vi "Write System Error To DB.vi"(8 "error in (no error)":errorcluster, 10 "Error_Payload":T1, 11 "Refnum in":T2) -> (0 "error out":errorcluster, 3 "Refnum out":T2)   [LabVIEW 2026, in "Database.lvlib"]
uses:
  Database.lvlib
  <vilib>/addons/database/Connection.llb/Conn ObjectReference.ctl
  controls/Diagnostics/Error_Payload.ctl
  <vilib>/addons/database/Connection.llb/Conn Execute.vi
  <vilib>/addons/database/Recordset.llb/Rec Destroy - Connection.vi
  <vilib>/addons/database/NI_Database_API.lvlib
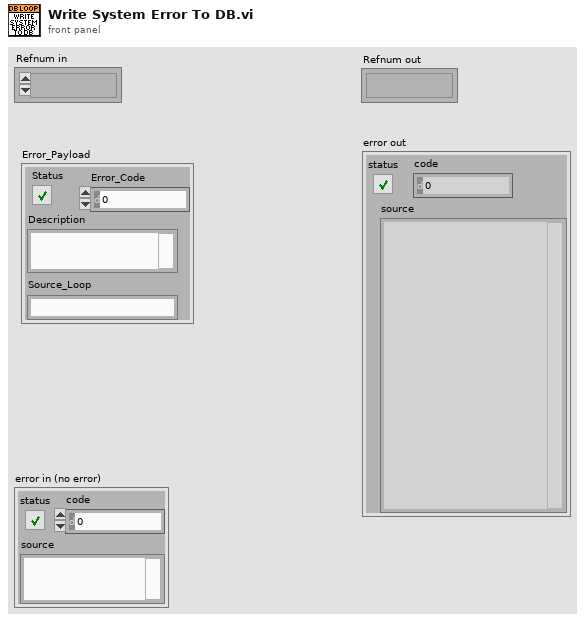
[diagram p1: front panel]
types:
  T1 = typedef "Error_Payload.ctl" = cluster{"status":bool, "error_code":i32, "description":string, "source_loop":string}
  T2 = typedef "NI_Database_API.lvlib/Conn ObjectReference.ctl" = refnum<k1>
  T3 = typedef "NI_Database_API.lvlib/Rec ObjectReference.ctl" = refnum<k1>
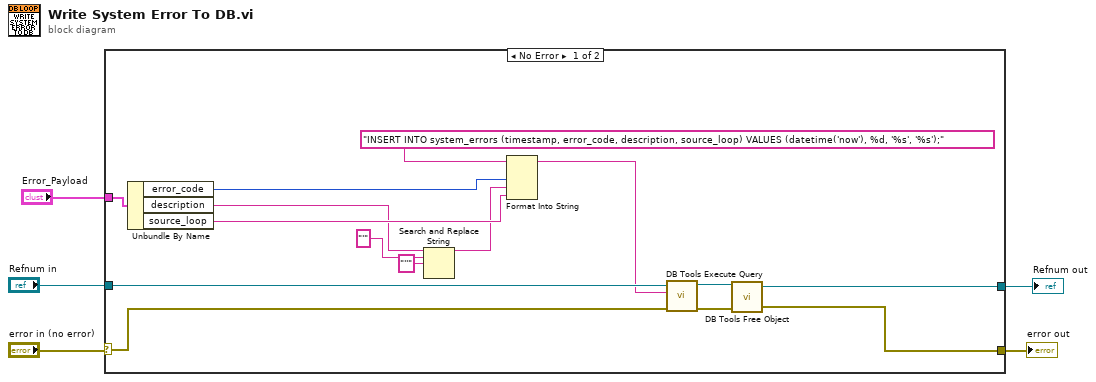
[diagram p0: block diagram]
diagram:
  n1 = case shown="No Error" "error in (no error)" {
    selector: "error in (no error)" -> [w18 w22]
    tunnel: [w16 w22] -> w5
    tunnel: [w17 w21] -> w4
    tunnel: "Refnum in" -> [w19 w21]
    tunnel: "Error_Payload" -> [w20 _]
    frame No Error {
      n2 = Unbundle By Name(w20) -> ("error_code"=w7:i32, "description"=w10:string, "source_loop"=w11:string)
      n3 = Search and Replace String(input string=w10, search string="'" ("format string"), replace string="''" ("replace string (\"\")")) -> (result string=w6:string)  [unwired: 5 in, 3 out]
      n4 = Format Into String(format string="INSERT INTO system_errors (timestamp, error_code, description, source_loop) VALUES (datetime('now'), %d, '%s', '%s');", w7, w6, w11) -> (resulting string=w14:string)  [unwired: 2 in, 1 out]
      n5 = call-poly <vilib>:"DB Tools Execute Query.vi"("error in (no error)"=w18, "SQL query"=w14, "connection reference"=w19) -> ("error out"=w13:errorcluster, "recordset reference"=w12:T3)  [unwired: 5 in]
      n6 = call-poly <vilib>:"DB Tools Free Object.vi"("error in (no error)"=w13, "recordset reference"=w12) -> ("error out"=w16:errorcluster, "connection reference"=w17:T2)  [unwired: 8 in]
    }
    frame Error {
    }
  }
  "error out" <- w5
  "Refnum out" <- w4
